vi "Initialize Network Comm Global.vi"(8 "error in (no error)":errorcluster) -> (0 "error out":errorcluster {"code" min=0 max=0}, 3 "Ref":T1)   [LabVIEW 2013, in "Instrument Addon Engine.lvlib" / "Network Common API.lvlib"]
uses:
  Network Common API.lvlib
  Network Comm Global Ref.ctl
  <userlib>/STM/Connection Manager/TCP/stm_TCPConnectionMethod.ctl
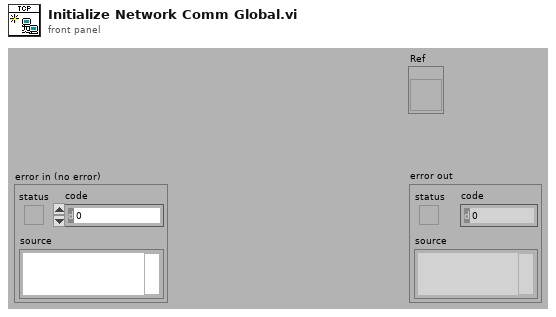
[diagram p1: front panel]
types:
  T1 = typedef "Instrument Addon Engine.lvlib/Network Common API.lvlib/Network Comm Global Ref.ctl" = refnum<vi>
  T2 = typedef "stm_TCPConnectionMethod.ctl" = enum16{"Initialize", "Add Connection", "Set Properties", "Get Connection(s)", "Remove Connection", "Remove All Connections", "Get Connection Count"}
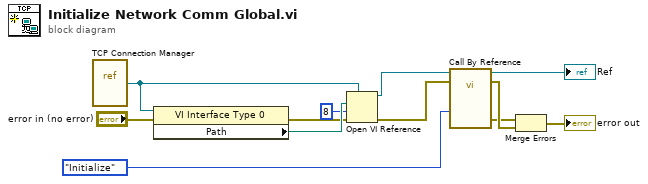
[diagram p0: block diagram]
diagram:
  n1 = vi-ref "TCP Connection Manager.vi"() -> (w7:refnum<vi>)
  n2 = property class="VI Interface Type 0"(reference=w7, error in="error in (no error)") -> (error out=w10:errorcluster, "Path"=w12:path)  [unwired: 1 out]
  n3 = Open VI Reference(type specifier VI Refnum (for type only)=w7, vi path=w12, options=8, error in (no error)=w10) -> (vi reference=w6:refnum<vi>, error out=w5:errorcluster)  [unwired: 2 in]
  n4 = call-by-ref "?"(reference=w6, error in=w5, "Method"=stm_TCPConnectionMethod."Initialize") -> (reference out=→"Ref":refnum<vi>, error out=w4:errorcluster, 0:"error out"=w3:errorcluster)  [unwired: 5 in, 5 out]
  n5 = Merge Errors(w3, w4) -> (→"error out":errorcluster)
